vi "ReadBinaryFile.vi"(7 "error in":errorcluster, 10 "file path (use dialog)":path) -> (0 "error out":errorcluster, 3 "byte array":u8[](array[numeric]))   [LabVIEW 2015]
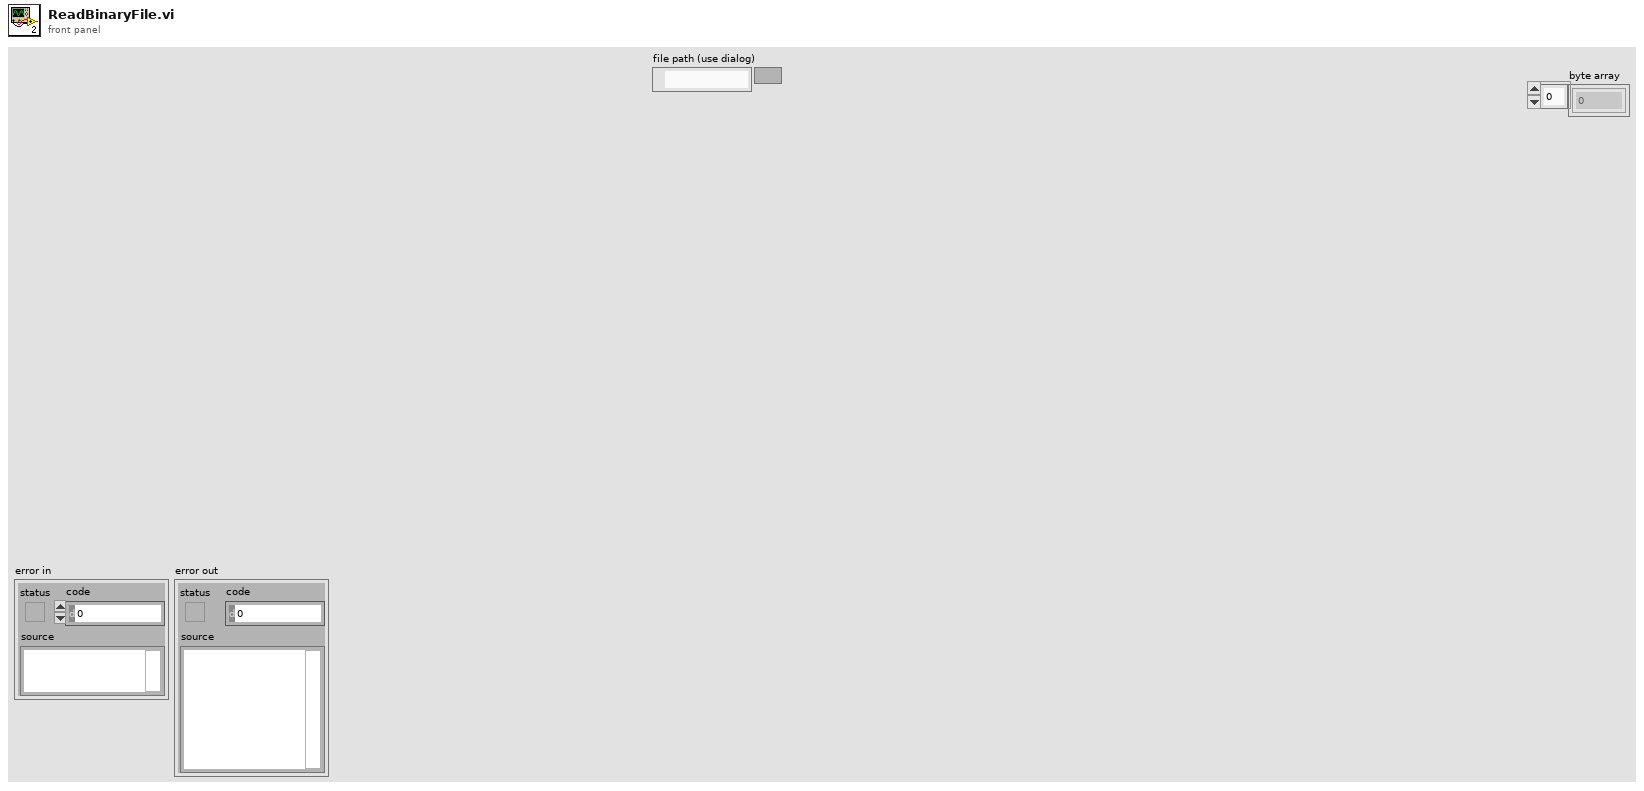
[diagram p1: front panel]
types:
  T1 = enum16{"open", "replace", "create", "open or create", "replace or create", "replace or create with confirmation"}
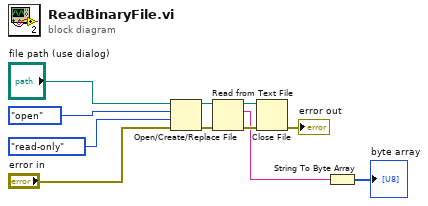
[diagram p0: block diagram]
diagram:
  n1 = Open/Create/Replace File(file path (use dialog)="file path (use dialog)", error in="error in", operation (0:open)=T1."open", access (0:read/write)=enum16{"read/write", "read-only", "write-only"}."read-only") -> (refnum out=w11:refnum<file>, error out=w10:errorcluster)  [unwired: 2 in, 1 out]
  n2 = Read from Text File(file (use dialog)=w11, error in=w10) -> (refnum out=w7:refnum<file>, text=w2:string, error out=w8:errorcluster)  [unwired: 2 in, 1 out]
  n3 = Close File(refnum=w7, error in=w8) -> (error out=→"error out":errorcluster)  [unwired: 1 out]
  n4 = String To Byte Array(string=w2) -> (unsigned byte array=→"byte array":u8[])
